vi "cosnowego2.vi"(11 "Waveform":waveform(dbl)) -> (1 "Numeric":dbl, 2 "Numeric 2":i32, 3 "As z A(1)":cdb[](array[numeric]), 4 "wykres 2":waveform(dbl), 5 "As":cdb[](array[numeric]), 6 "df":dbl, 7 "N2":dbl)   [LabVIEW 2025]
uses:
  <vilib>/Analysis/NI_AALPro.lvlib
  <vilib>/Analysis/2dsp.llb/Real FFT.vi
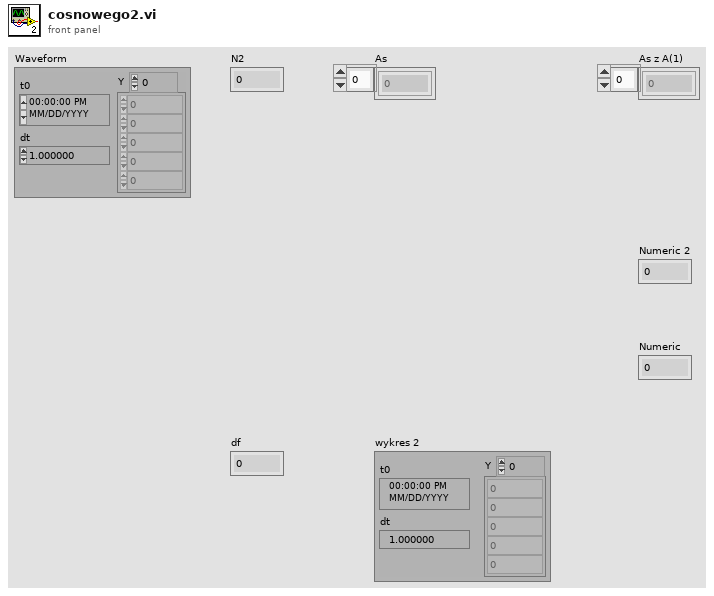
[diagram p1: front panel]
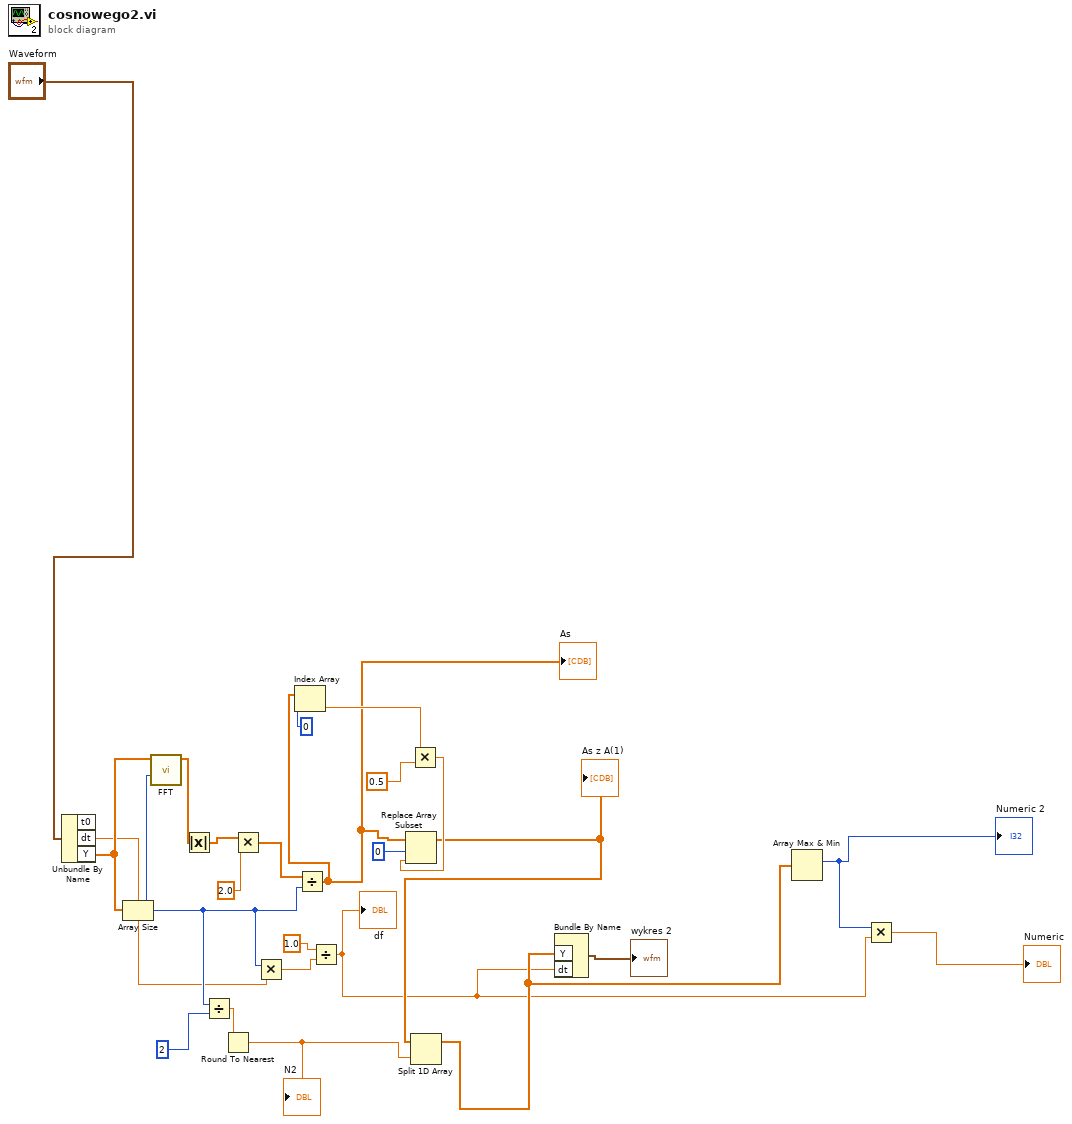
[diagram p0: block diagram]
diagram:
  n1 = Unbundle By Name("Waveform") -> ("dt"=w8:dbl, "Y"=w24:dbl[])  [unwired: 1 out]
  n2 = Array Size(array=w24) -> (size(s)=w19:i32)
  n3 = call-poly <vilib>:"FFT.vi"("FFT size"=w19, "X"=w24) -> ("FFT {X}"=w11:cdb[])  [unwired: 8 in, 1 out]
  n4 = Absolute Value(x=w11) -> (abs(x)=w10:dbl[])
  n5 = Divide(x=w19, y=2) -> (x/y=w17:dbl)
  n6 = Round To Nearest(number=w17) -> (nearest integer value=w6:dbl)
  "N2" <- w6
  n7 = Multiply(x=w10, y=2.0) -> (x*y=w22:dbl[])
  n8 = Multiply(x=w19, y=w8) -> (x*y=w20:dbl)
  n9 = Divide(x=w22, y=w19) -> (x/y=w12:dbl[])
  "As" <- w12
  n10 = Index Array(array=w12, index=0) -> (element=w14:dbl)
  n11 = Divide(x=1.0, y=w20) -> (x/y=w2:dbl)
  "df" <- w2
  n12 = Multiply(x=w14, y=0.5) -> (x*y=w13:dbl)
  n13 = Replace Array Subset(array=w12, new element=w13, index=0) -> (w7:dbl[])
  "As z A(1)" <- w7
  n14 = Split 1D Array(array=w7, index=w6) -> (first subarray=w4:dbl[])  [unwired: 1 out]
  n15 = Bundle By Name("Y"=w4, "dt"=w2) -> (→"wykres 2":waveform(dbl))  [unwired: 1 in]
  n16 = Array Max & Min(array=w4) -> (max index (indices)=w3:i32)  [unwired: 3 out]
  "Numeric 2" <- w3
  n17 = Multiply(x=w3, y=w2) -> (x*y=→"Numeric":dbl)
